vi "Example Tractor Lights 1.vi"() -> ()   [LabVIEW 2014]
panel:
  in  "Error In":errorcluster
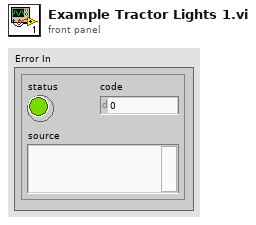
[diagram p1: front panel]
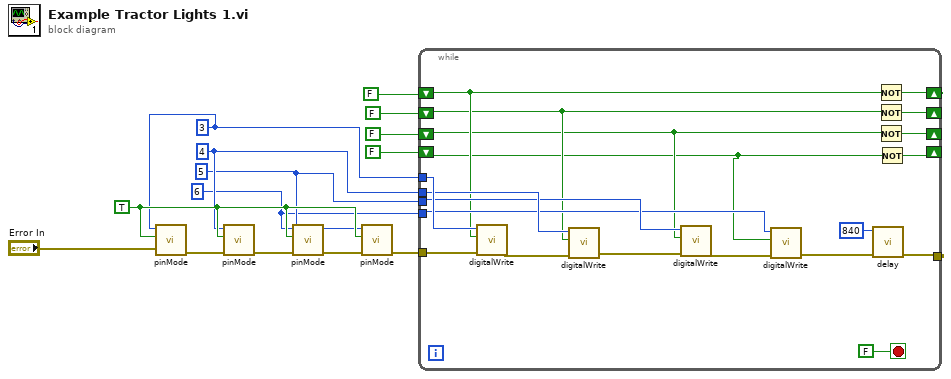
[diagram p0: block diagram]
diagram:
  w4 = 3 ("pin number")
  w3 = 4 ("pin number")
  w2 = 5 ("pin number")
  w1 = 6 ("pin number")
  w11 = TRUE ("output?")
  n1 = call <vilib>:"pinMode.vi"("Error In"="Error In", "output?"=w11, "pin number"=w4) -> ("Error Out"=w14:errorcluster)  [unwired: 8 in]
  n2 = call <vilib>:"pinMode.vi"("Error In"=w14, "output?"=w11, "pin number"=w3) -> ("Error Out"=w13:errorcluster)  [unwired: 8 in]
  n3 = call <vilib>:"pinMode.vi"("Error In"=w13, "output?"=w11, "pin number"=w2) -> ("Error Out"=w12:errorcluster)  [unwired: 8 in]
  n4 = call <vilib>:"pinMode.vi"("Error In"=w12, "output?"=w11, "pin number"=w1) -> ("Error Out"=w9:errorcluster)  [unwired: 8 in]
  n5 = while {
    tunnel: w9 -> [w34]
    shift-right: [w33] -> _
    shift-left: FALSE ("output?") -> [w22]
    shift-right: [w32] -> _
    shift-left: FALSE ("output?") -> [w21]
    shift-right: [w31] -> _
    shift-left: FALSE ("output?") -> [w20]
    shift-right: [w30] -> _
    shift-left: FALSE ("output?") -> [w19]
    tunnel: w4 -> [w26]
    tunnel: w3 -> [w25]
    tunnel: w2 -> [w24]
    tunnel: w1 -> [w23]
    tunnel: [w16] -> _
    stop <- FALSE stop-if-true
    n6 = call <vilib>:"digitalWrite.vi"("Error In"=w34, "value"=w22, "pin number"=w26) -> ("Error Out"=w27:errorcluster)  [unwired: 8 in]
    n7 = call <vilib>:"digitalWrite.vi"("Error In"=w27, "value"=w21, "pin number"=w25) -> ("Error Out"=w28:errorcluster)  [unwired: 8 in]
    n8 = call <vilib>:"digitalWrite.vi"("Error In"=w28, "value"=w20, "pin number"=w24) -> ("Error Out"=w29:errorcluster)  [unwired: 8 in]
    n9 = call <vilib>:"digitalWrite.vi"("Error In"=w29, "value"=w19, "pin number"=w23) -> ("Error Out"=w17:errorcluster)  [unwired: 8 in]
    n10 = call <vilib>:"delay.vi"("Error In"=w17, "time (ms)"=840) -> ("Error Out"=w16:errorcluster)  [unwired: 9 in]
    n11 = Not(x=w22) -> (.not. x?=w33:bool)
    n12 = Not(x=w21) -> (.not. x?=w32:bool)
    n13 = Not(x=w20) -> (.not. x?=w31:bool)
    n14 = Not(x=w19) -> (.not. x?=w30:bool)
  }
